vi "readSDOU32.vi"(6 "interface object in":refnum<k20>, 8 "error in (no error)":errorcluster, 9 "subIndex":u8, 10 "objectIndex":u16, 11 "MotorController in":refnum<class "MotorController.lvclass">) -> (0 "error out":errorcluster, 1 "interface object out":refnum<k20>, 2 "output":u32, 3 "MotorController out":refnum<class "MotorController.lvclass">)   [LabVIEW 2017, in "MotorController.lvclass"]
uses:
  MotorController.lvclass
  MotorController.lvclass/MotorController.ctl
  <vilib>/CANopenLib/CANOPEN.llb/CANopen SDO Create.vi
  <vilib>/CANopenLib/CANOPEN.llb/CANopen SDO Read [U32].vi
  <vilib>/CANopenLib/CANOPEN.llb/CANopen SDO Close.vi
panel:
  out "completion code":u32 format="%.0x"
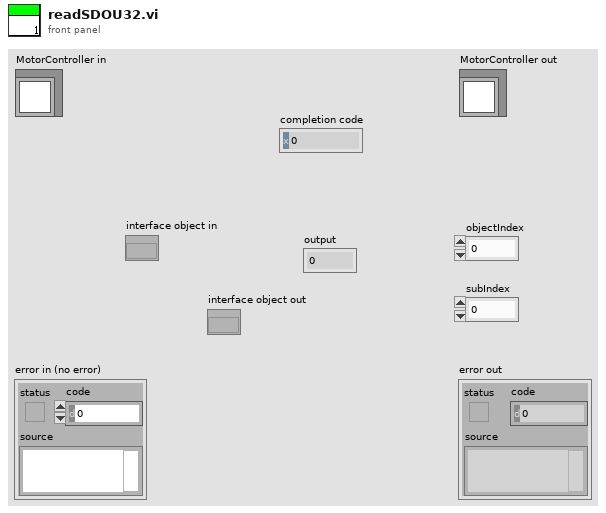
[diagram p1: front panel]
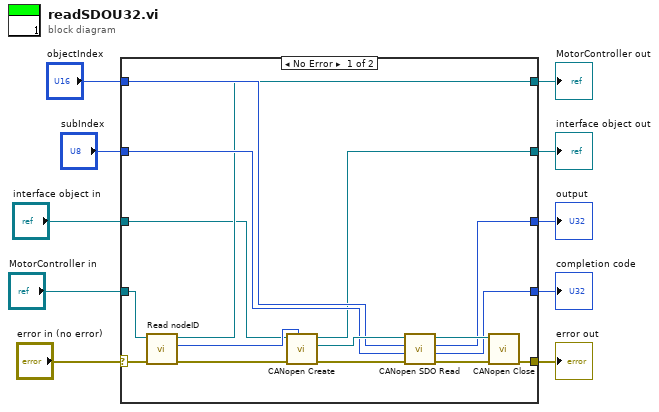
[diagram p0: block diagram]
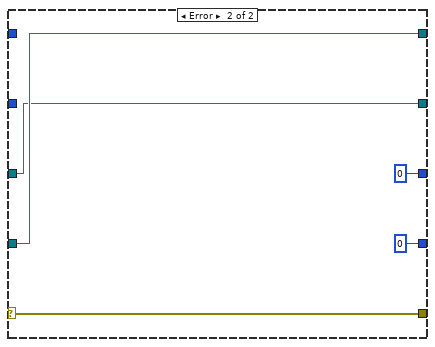
[diagram p2: hidden frame]
diagram:
  n1 = case shown="No Error" "error in (no error)" {
    selector: "error in (no error)" -> [w15 w31]
    tunnel: [w13 w31] -> w6
    tunnel: [w17 w30] -> w7
    tunnel: "MotorController in" -> [w16 w30]
    tunnel: [w20 u32 0 ("U32 data")] -> w8
    tunnel: "subIndex" -> [w19 _]
    tunnel: "objectIndex" -> [w18 _]
    tunnel: "interface object in" -> [w14 w28]
    tunnel: [w12 w28] -> w2
    tunnel: [w11 u32 0 ("completion code")] -> w1
    frame No Error {
      n2 = call "Read nodeID.vi"("error in (no error)"=w15, "MotorController in"=w16) -> ("error out"=w25:errorcluster, "nodeID"=w26:u8, "MotorController out"=w17:refnum<class "MotorController.lvclass">)  [unwired: 7 in]
      n3 = call-poly <vilib>:"CANopen Create.vi"("node-ID"=w26, "error in (no error)"=w25, "interface object in"=w14) -> ("error out"=w24:errorcluster, "SDO object out"=w23:refnum<k20>, "interface object out"=w12:refnum<k20>)  [unwired: 6 in]
      n4 = call-poly <vilib>:"CANopen SDO Read.vi"("error in (no error)"=w24, "object sub-index (0)"=w19, "object index"=w18, "SDO object in"=w23) -> ("error out"=w21:errorcluster, "completion code"=w11:u32, "U32 data"=w20:u32, "SDO object out"=w22:refnum<k20>)  [unwired: 4 in]
      n5 = call-poly <vilib>:"CANopen Close.vi"("error in (no error)"=w21, "SDO object in"=w22) -> ("error out"=w13:errorcluster)  [unwired: 9 in]
    }
    frame Error {
    }
  }
  "error out" <- w6
  "MotorController out" <- w7
  "output" <- w8
  "interface object out" <- w2
  "completion code" <- w1
